vi "(Instrl) Chamber.vi"(7 "State":T1, 8 "error in (no error)":errorcluster caption="에러 입력(에러 없음)", 10 "Taget Temp":u16, 11 "Com":refnum<visa-resource-name> caption="VISA 리소스 이름") -> (0 "error out":errorcluster caption="에러 출력", 1 "Run ?":bool, 2 "Target Temp":dbl, 3 "Chamber Temp":dbl)   [LabVIEW 2017]
uses:
  Controls/(Ctrl) State_Chamber.ctl
  d33bea22-d172-46f5-8023-11f0f0edf04c.vi
  4e8498e9-99a5-4009-ae3f-178909532f49.vi
  1dfa9a5f-52c3-4c21-9b15-0f595ffaef15.vi
  832b1939-2673-4a84-9c7a-3456cb382369.vi
  1d00543b-5e07-4994-bebe-18b56b2cc428.vi
  badd6b8b-c736-49e5-b97b-2faf3af165ed.vi
  e5d39b2c-7c74-48f6-a464-7171ab566bb8.vi
  0904d720-0f40-4f53-a6e3-23163ff1973b.vi
  8535f138-c1eb-4e0f-a714-550ec1784386.vi
  a9bdc2db-8e9a-46e3-b93c-271c825e978d.vi
  f088d943-c508-4480-85fa-39f76ade122a.vi
  ab44e7ac-ed16-4d77-bafb-c9659d96e42c.vi
  <vilib>/Instr/_visa.llb/VISA Configure Serial Port (Instr).vi
panel:
  out "버퍼 읽기":string
  out "Read Data":string
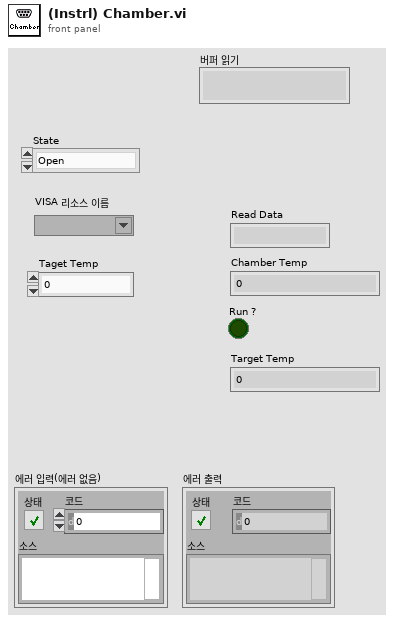
[diagram p1: front panel]
types:
  T1 = typedef "(Ctrl) State_Chamber.ctl" = enum16{"Open", "Rx : Temp", "Rx : Target Temp", "Rx : State", "Tx : ON-OFF", "Tx : Target Temp", "Tx : Time Set", "Close"}
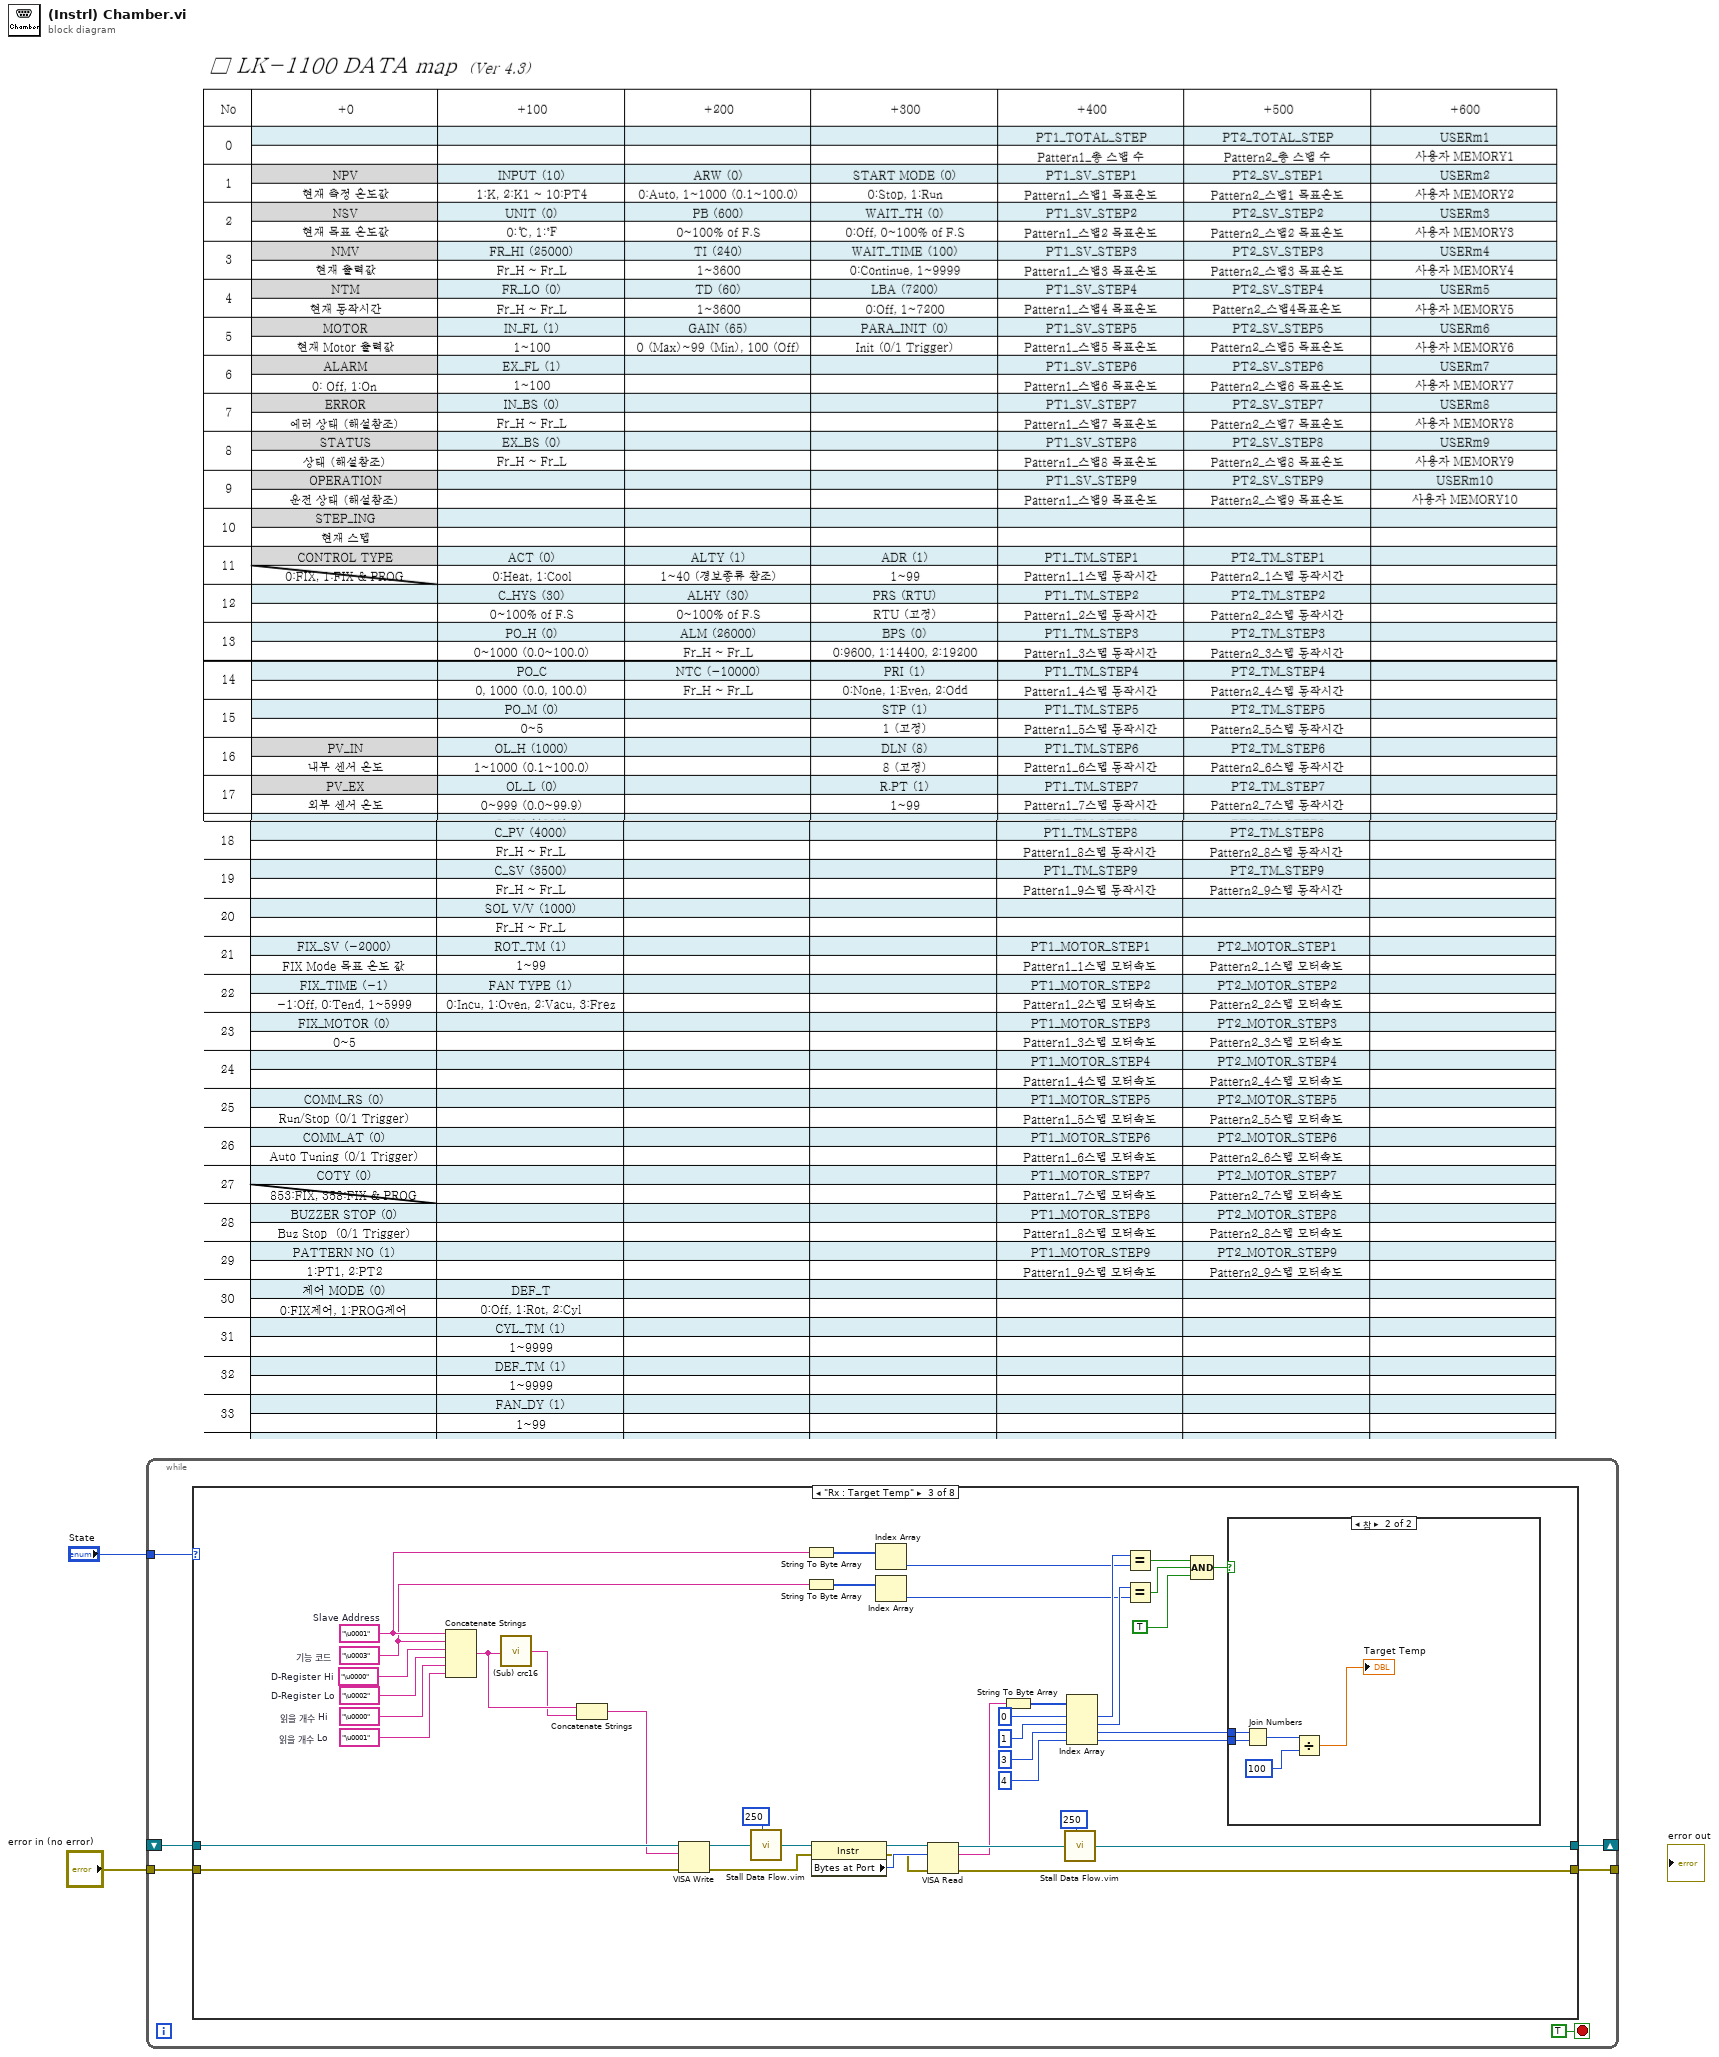
[diagram p0: block diagram]
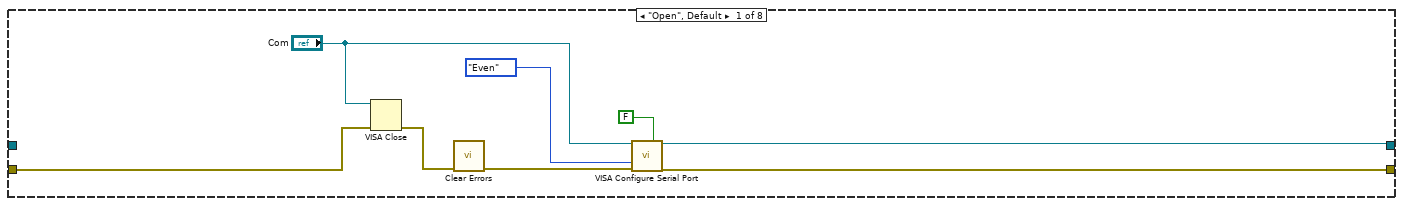
[diagram p2: hidden frame]
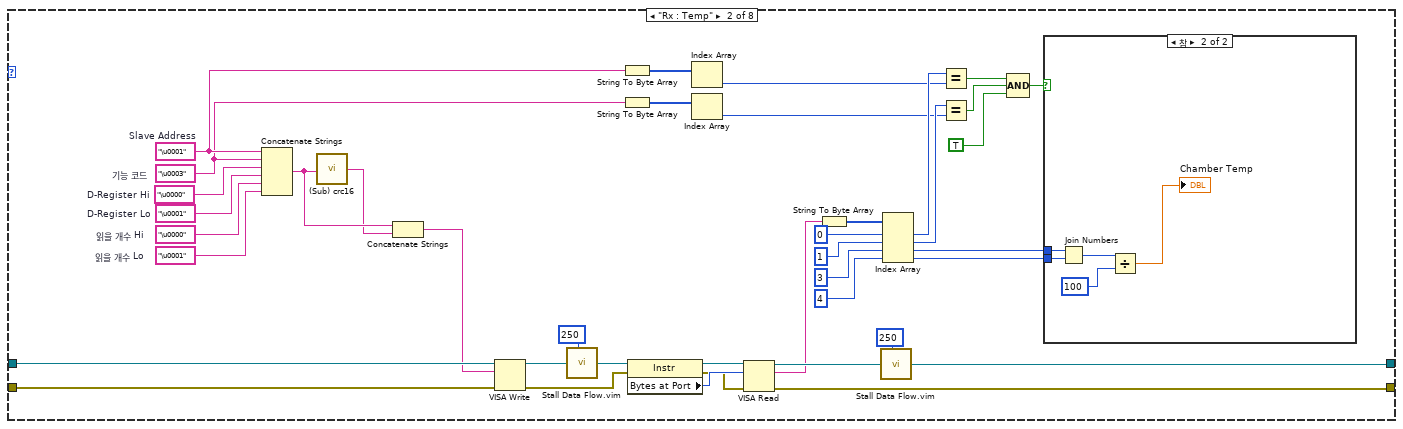
[diagram p3: hidden frame]
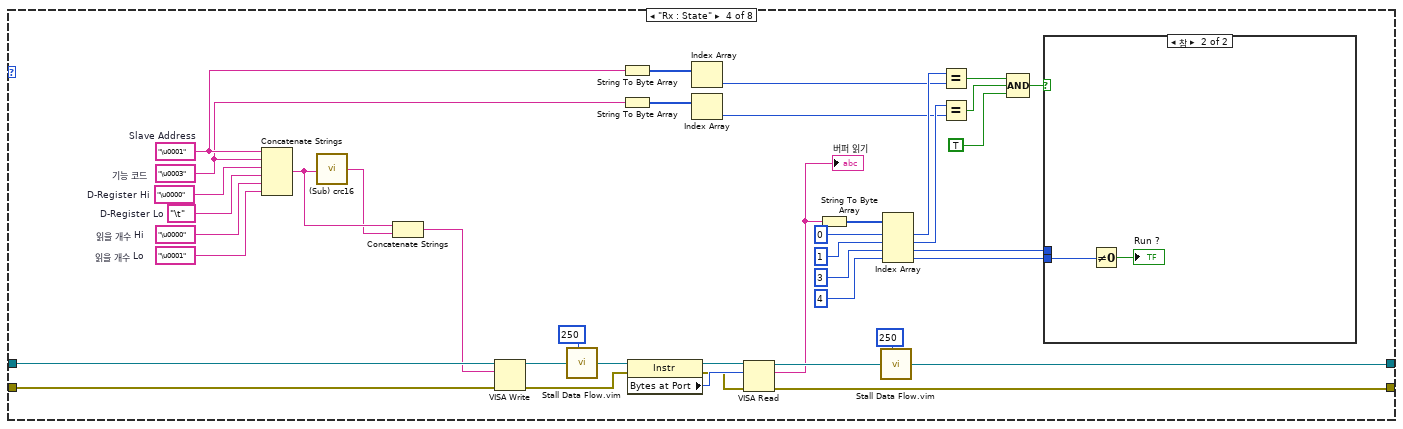
[diagram p6: hidden frame]
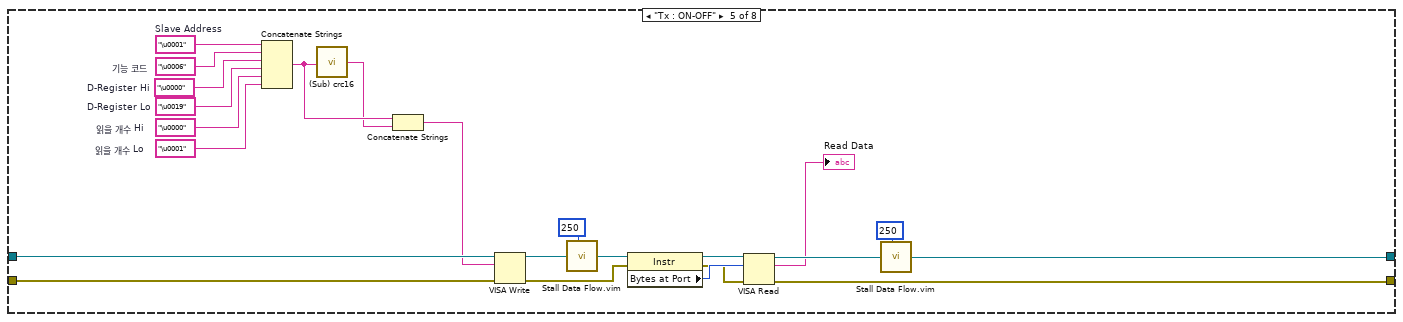
[diagram p8: hidden frame]
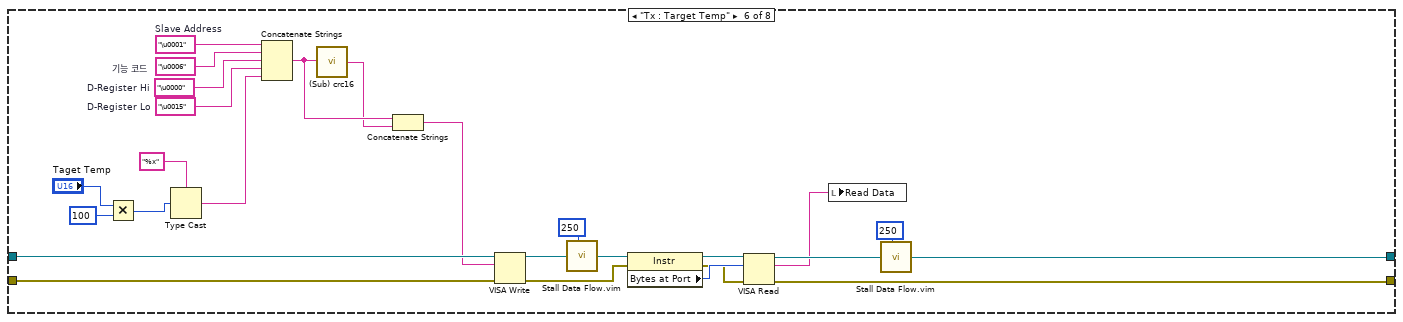
[diagram p9: hidden frame]
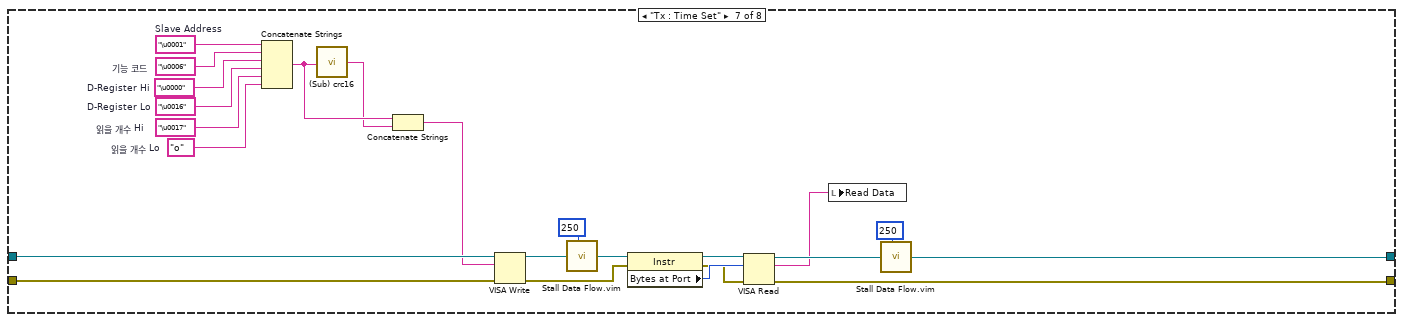
[diagram p10: hidden frame]
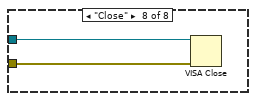
[diagram p11: hidden frame]
diagram:
  n1 = while {
    tunnel: "State" -> [w7]
    tunnel: "error in (no error)" -> [w6]
    shift-right: [w5] -> _
    shift-left: _ -> [w3]
    tunnel: [w4] -> _
    stop <- TRUE stop-if-true
    n2 = case shown="\"Rx : Target Temp\"" w7 {
      tunnel: w6 -> [w16 w55 w100 w145 w170 w196 w219 w221]
      tunnel: [w13 w38 w83 w128 w153 w181 w203 _] -> w5
      tunnel: [w12 w39 w84 w129 w154 w182 w204 _] -> w4
      tunnel: w3 -> [_ w56 w101 w146 w171 w197 w220 w222]
      frame "Open", Default {
        n3 = VISA Close(VISA resource name="Com", error in (no error)=w16) -> (error out=w10:errorcluster)
        n4 = call <vilib>:"Clear Errors.vi"("error in (no error)"=w10) -> ("error out"=w9:errorcluster)  [unwired: 5 in, 1 out]
        n5 = call-poly "VISA Configure Serial Port"("VISA resource name"="Com", "Enable Termination\nChar (T)"=FALSE ("Enable Termination\nChar (T)"), "parity (0:none)"=enum16{"None", "Odd", "Even", "Mark", "Space"}."Even", "error in (no error)"=w9) -> ("VISA resource name out"=w13:refnum<visa-resource-name>, "error out"=w12:errorcluster)  [unwired: 10 in]
      }
      frame "Rx : Temp" {
        w51 = "\u0001"  # 읽을 개수 Lo
        w52 = "\u0000"  # 읽을 개수 Hi
        w53 = "\u0001"  # D-Register Lo
        w54 = "\u0000"  # D-Register Hi
        w31 = "\u0003"  # 기능 코드
        w34 = "\u0001"  # Slave Address
        n6 = Concatenate Strings(w34, w31, w54, w53, w52, w51) -> (w50:string)
        n7 = call "(Sub) crc16.vi"("message"=w50) -> ("CRC16"=w49:string)  [unwired: 4 in]
        n8 = Concatenate Strings(w50, w49) -> (w48:string)
        n9 = VISA Write(VISA resource name=w56, write buffer=w48, error in (no error)=w55) -> (VISA resource name out=w45:refnum<visa-resource-name>, error out=w46:errorcluster)  [unwired: 1 out]
        n10 = call "Stall Data Flow.vim"("value in"=w45, "milliseconds to wait"=u32 250) -> ("value out"=w44:refnum<visa-resource-name>)  [unwired: 1 out]
        n11 = String To Byte Array(string=w34) -> (unsigned byte array=w33:u8[])
        n12 = String To Byte Array(string=w31) -> (unsigned byte array=w32:u8[])
        n13 = property class="Instr"(reference=w44, error in=w46) -> (reference out=w43:refnum<visa-resource-name>, error out=w41:errorcluster, "Bytes at Port"=w42:u32)
        n14 = Index Array(array=w33) -> (element=w28:u8)  [unwired: 1 in]
        n15 = Index Array(array=w32) -> (element=w26:u8)  [unwired: 1 in]
        n16 = VISA Read(VISA resource name=w43, byte count=w42, error in (no error)=w41) -> (VISA resource name out=w40:refnum<visa-resource-name>, read buffer=w36:string, error out=w39:errorcluster)  [unwired: 1 out]
        n17 = String To Byte Array(string=w36) -> (unsigned byte array=w35:u8[])
        n18 = call "Stall Data Flow.vim"("value in"=w40, "milliseconds to wait"=u32 250) -> ("value out"=w38:refnum<visa-resource-name>)  [unwired: 1 out]
        n19 = Index Array(array=w35, index #1=0 ("인덱스"), index #2=1 ("인덱스"), index #3=3 ("인덱스"), index #4=4 ("인덱스")) -> (element #1=w29:u8, element #2=w27:u8, element #3=w18:u8, element #4=w17:u8)
        n20 = Equal?(x=w29, y=w28) -> (x = y?=w25:bool)
        n21 = Equal?(x=w27, y=w26) -> (x = y?=w24:bool)
        n22 = Compound Arithmetic op=AND(w25, w24, TRUE) -> (w22:bool)
        n23 = case shown="참" w22 {
          tunnel: w18 -> [_ w61]
          tunnel: w17 -> [_ w60]
          frame False {
          }
          frame True {
            n24 = Join Numbers(hi=w61, lo=w60) -> ((hi.lo)=w59:u16)
            n25 = Divide(x=w59, y=u16 100) -> (x/y=→"Chamber Temp":dbl)
          }
        }
      }
      frame "Rx : Target Temp" {
        w96 = "\u0001"  # 읽을 개수 Lo
        w97 = "\u0000"  # 읽을 개수 Hi
        w98 = "\u0002"  # D-Register Lo
        w99 = "\u0000"  # D-Register Hi
        w76 = "\u0003"  # 기능 코드
        w79 = "\u0001"  # Slave Address
        n26 = Concatenate Strings(w79, w76, w99, w98, w97, w96) -> (w95:string)
        n27 = call "(Sub) crc16.vi"("message"=w95) -> ("CRC16"=w94:string)  [unwired: 4 in]
        n28 = Concatenate Strings(w95, w94) -> (w93:string)
        n29 = VISA Write(VISA resource name=w101, write buffer=w93, error in (no error)=w100) -> (VISA resource name out=w90:refnum<visa-resource-name>, error out=w91:errorcluster)  [unwired: 1 out]
        n30 = call "Stall Data Flow.vim"("value in"=w90, "milliseconds to wait"=u32 250) -> ("value out"=w89:refnum<visa-resource-name>)  [unwired: 1 out]
        n31 = String To Byte Array(string=w79) -> (unsigned byte array=w78:u8[])
        n32 = String To Byte Array(string=w76) -> (unsigned byte array=w77:u8[])
        n33 = property class="Instr"(reference=w89, error in=w91) -> (reference out=w88:refnum<visa-resource-name>, error out=w86:errorcluster, "Bytes at Port"=w87:u32)
        n34 = Index Array(array=w78) -> (element=w73:u8)  [unwired: 1 in]
        n35 = Index Array(array=w77) -> (element=w71:u8)  [unwired: 1 in]
        n36 = VISA Read(VISA resource name=w88, byte count=w87, error in (no error)=w86) -> (VISA resource name out=w85:refnum<visa-resource-name>, read buffer=w81:string, error out=w84:errorcluster)  [unwired: 1 out]
        n37 = String To Byte Array(string=w81) -> (unsigned byte array=w80:u8[])
        n38 = call "Stall Data Flow.vim"("value in"=w85, "milliseconds to wait"=u32 250) -> ("value out"=w83:refnum<visa-resource-name>)  [unwired: 1 out]
        n39 = Index Array(array=w80, index #1=0 ("인덱스"), index #2=1 ("인덱스"), index #3=3 ("인덱스"), index #4=4 ("인덱스")) -> (element #1=w74:u8, element #2=w72:u8, element #3=w63:u8, element #4=w62:u8)
        n40 = Equal?(x=w74, y=w73) -> (x = y?=w70:bool)
        n41 = Equal?(x=w72, y=w71) -> (x = y?=w69:bool)
        n42 = Compound Arithmetic op=AND(w70, w69, TRUE) -> (w67:bool)
        n43 = case shown="참" w67 {
          tunnel: w63 -> [_ w106]
          tunnel: w62 -> [_ w105]
          frame False {
          }
          frame True {
            n44 = Join Numbers(hi=w106, lo=w105) -> ((hi.lo)=w104:u16)
            n45 = Divide(x=w104, y=u16 100) -> (x/y=→"Target Temp":dbl)
          }
        }
      }
      frame "Rx : State" {
        w141 = "\u0001"  # 읽을 개수 Lo
        w142 = "\u0000"  # 읽을 개수 Hi
        w143 = "\t"  # D-Register Lo
        w144 = "\u0000"  # D-Register Hi
        w121 = "\u0003"  # 기능 코드
        w124 = "\u0001"  # Slave Address
        n46 = Concatenate Strings(w124, w121, w144, w143, w142, w141) -> (w140:string)
        n47 = call "(Sub) crc16.vi"("message"=w140) -> ("CRC16"=w139:string)  [unwired: 4 in]
        n48 = Concatenate Strings(w140, w139) -> (w138:string)
        n49 = VISA Write(VISA resource name=w146, write buffer=w138, error in (no error)=w145) -> (VISA resource name out=w135:refnum<visa-resource-name>, error out=w136:errorcluster)  [unwired: 1 out]
        n50 = call "Stall Data Flow.vim"("value in"=w135, "milliseconds to wait"=u32 250) -> ("value out"=w134:refnum<visa-resource-name>)  [unwired: 1 out]
        n51 = String To Byte Array(string=w124) -> (unsigned byte array=w123:u8[])
        n52 = String To Byte Array(string=w121) -> (unsigned byte array=w122:u8[])
        n53 = property class="Instr"(reference=w134, error in=w136) -> (reference out=w133:refnum<visa-resource-name>, error out=w131:errorcluster, "Bytes at Port"=w132:u32)
        n54 = Index Array(array=w123) -> (element=w118:u8)  [unwired: 1 in]
        n55 = Index Array(array=w122) -> (element=w116:u8)  [unwired: 1 in]
        n56 = VISA Read(VISA resource name=w133, byte count=w132, error in (no error)=w131) -> (VISA resource name out=w130:refnum<visa-resource-name>, read buffer=w126:string, error out=w129:errorcluster)  [unwired: 1 out]
        "버퍼 읽기" <- w126
        n57 = String To Byte Array(string=w126) -> (unsigned byte array=w125:u8[])
        n58 = call "Stall Data Flow.vim"("value in"=w130, "milliseconds to wait"=u32 250) -> ("value out"=w128:refnum<visa-resource-name>)  [unwired: 1 out]
        n59 = Index Array(array=w125, index #1=0 ("인덱스"), index #2=1 ("인덱스"), index #3=3 ("인덱스"), index #4=4 ("인덱스")) -> (element #1=w119:u8, element #2=w117:u8, element #3=w108:u8, element #4=w107:u8)
        n60 = Equal?(x=w119, y=w118) -> (x = y?=w115:bool)
        n61 = Equal?(x=w117, y=w116) -> (x = y?=w114:bool)
        n62 = Compound Arithmetic op=AND(w115, w114, TRUE) -> (w112:bool)
        n63 = case shown="참" w112 {
          tunnel: w108 -> [_ _]
          tunnel: w107 -> [_ w148]
          frame False {
          }
          frame True {
            n64 = Not Equal To 0?(x=w148) -> (x != 0?=→"Run ?":bool)
          }
        }
      }
      frame "Tx : ON-OFF" {
        w166 = "\u0001"  # 읽을 개수 Lo
        w167 = "\u0000"  # 읽을 개수 Hi
        w168 = "\u0019"  # D-Register Lo
        w169 = "\u0000"  # D-Register Hi
        w150 = "\u0006"  # 기능 코드
        w151 = "\u0001"  # Slave Address
        n65 = Concatenate Strings(w151, w150, w169, w168, w167, w166) -> (w165:string)
        n66 = call "(Sub) crc16.vi"("message"=w165) -> ("CRC16"=w164:string)  [unwired: 4 in]
        n67 = Concatenate Strings(w165, w164) -> (w163:string)
        n68 = VISA Write(VISA resource name=w171, write buffer=w163, error in (no error)=w170) -> (VISA resource name out=w160:refnum<visa-resource-name>, error out=w161:errorcluster)  [unwired: 1 out]
        n69 = call "Stall Data Flow.vim"("value in"=w160, "milliseconds to wait"=u32 250) -> ("value out"=w159:refnum<visa-resource-name>)  [unwired: 1 out]
        n70 = property class="Instr"(reference=w159, error in=w161) -> (reference out=w158:refnum<visa-resource-name>, error out=w156:errorcluster, "Bytes at Port"=w157:u32)
        n71 = VISA Read(VISA resource name=w158, byte count=w157, error in (no error)=w156) -> (VISA resource name out=w155:refnum<visa-resource-name>, read buffer=→"Read Data":string, error out=w154:errorcluster)  [unwired: 1 out]
        n72 = call "Stall Data Flow.vim"("value in"=w155, "milliseconds to wait"=u32 250) -> ("value out"=w153:refnum<visa-resource-name>)  [unwired: 1 out]
      }
      frame "Tx : Target Temp" {
        w194 = "\u0015"  # D-Register Lo
        w195 = "\u0000"  # D-Register Hi
        w178 = "\u0006"  # 기능 코드
        w179 = "\u0001"  # Slave Address
        n73 = Multiply(x="Taget Temp", y=u16 100) -> (x*y=w173:u16)
        n74 = Type Cast(type="%x" ("타입"), x=w173) -> (*(type *) &x=w174:string)
        n75 = Concatenate Strings(w179, w178, w195, w194, w174) -> (w193:string)
        n76 = call "(Sub) crc16.vi"("message"=w193) -> ("CRC16"=w192:string)  [unwired: 4 in]
        n77 = Concatenate Strings(w193, w192) -> (w191:string)
        n78 = VISA Write(VISA resource name=w197, write buffer=w191, error in (no error)=w196) -> (VISA resource name out=w188:refnum<visa-resource-name>, error out=w189:errorcluster)  [unwired: 1 out]
        n79 = call "Stall Data Flow.vim"("value in"=w188, "milliseconds to wait"=u32 250) -> ("value out"=w187:refnum<visa-resource-name>)  [unwired: 1 out]
        n80 = property class="Instr"(reference=w187, error in=w189) -> (reference out=w186:refnum<visa-resource-name>, error out=w184:errorcluster, "Bytes at Port"=w185:u32)
        n81 = VISA Read(VISA resource name=w186, byte count=w185, error in (no error)=w184) -> (VISA resource name out=w183:refnum<visa-resource-name>, read buffer=w177:string, error out=w182:errorcluster)  [unwired: 1 out]
        n82 = local write "Read Data"(w177) -> ()
        n83 = call "Stall Data Flow.vim"("value in"=w183, "milliseconds to wait"=u32 250) -> ("value out"=w181:refnum<visa-resource-name>)  [unwired: 1 out]
      }
      frame "Tx : Time Set" {
        w198 = "o"  # 읽을 개수 Lo
        w216 = "\u0017"  # 읽을 개수 Hi
        w217 = "\u0016"  # D-Register Lo
        w218 = "\u0000"  # D-Register Hi
        w200 = "\u0006"  # 기능 코드
        w201 = "\u0001"  # Slave Address
        n84 = Concatenate Strings(w201, w200, w218, w217, w216, w198) -> (w215:string)
        n85 = call "(Sub) crc16.vi"("message"=w215) -> ("CRC16"=w214:string)  [unwired: 4 in]
        n86 = Concatenate Strings(w215, w214) -> (w213:string)
        n87 = VISA Write(VISA resource name=w220, write buffer=w213, error in (no error)=w219) -> (VISA resource name out=w210:refnum<visa-resource-name>, error out=w211:errorcluster)  [unwired: 1 out]
        n88 = call "Stall Data Flow.vim"("value in"=w210, "milliseconds to wait"=u32 250) -> ("value out"=w209:refnum<visa-resource-name>)  [unwired: 1 out]
        n89 = property class="Instr"(reference=w209, error in=w211) -> (reference out=w208:refnum<visa-resource-name>, error out=w206:errorcluster, "Bytes at Port"=w207:u32)
        n90 = VISA Read(VISA resource name=w208, byte count=w207, error in (no error)=w206) -> (VISA resource name out=w205:refnum<visa-resource-name>, read buffer=w199:string, error out=w204:errorcluster)  [unwired: 1 out]
        n91 = local write "Read Data"(w199) -> ()
        n92 = call "Stall Data Flow.vim"("value in"=w205, "milliseconds to wait"=u32 250) -> ("value out"=w203:refnum<visa-resource-name>)  [unwired: 1 out]
      }
      frame "Close" {
        n93 = VISA Close(VISA resource name=w222, error in (no error)=w221) -> ()  [unwired: 1 out]
      }
    }
  }
